vi "Receive Message.vi"(6 "timeout in ms (-1)":i32=-1, 8 "error in (no error)":errorcluster, 11 "QueueMessageTransport in":refnum<class "QueueMessageTransport.lvclass">) -> (0 "error out":errorcluster, 2 "Q Element":refnum<class "IMessagePayload.lvclass">, 3 "QueueMessageTransport out":refnum<class "QueueMessageTransport.lvclass">)   [LabVIEW 2016, in "QueueMessageTransport.lvclass"]
uses:
  QueueMessageTransport.lvclass
  IMessagePayload/IMessagePayload.lvclass
  QMHMessagePayload/QMHMessagePayload.lvclass
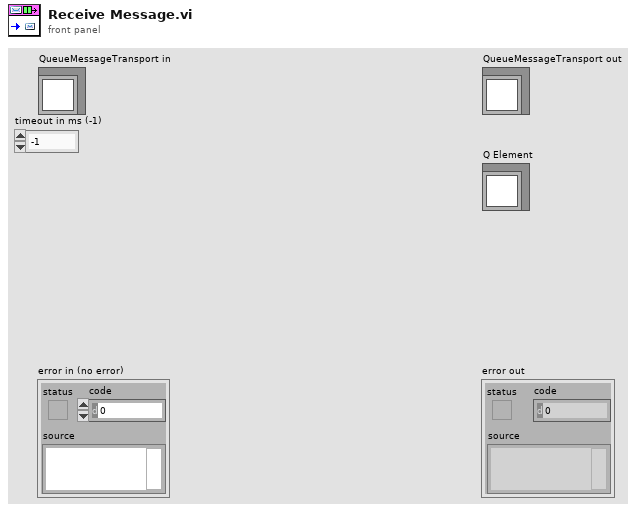
[diagram p1: front panel]
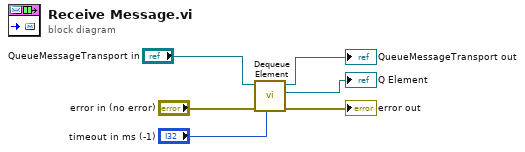
[diagram p0: block diagram]
diagram:
  n1 = call "Dequeue Element.vi"("timeout in ms (-1)"="timeout in ms (-1)", "error in"="error in (no error)", "QueueMessageTransport in"="QueueMessageTransport in") -> ("error out"=→"error out":errorcluster, "Q Element"=→"Q Element":refnum<class "IMessagePayload.lvclass">, "QueueMessageTransport out"=→"QueueMessageTransport out":refnum<class "QueueMessageTransport.lvclass">)  [unwired: 6 in]
